vi "ESC controller ramped.vi"(1 "Don't Wait":bool, 2 "Error In":errorcluster, 3 "Output %":sgl min=0 max=100) -> (0 "Error out":errorcluster)   [LabVIEW 2021]
uses:
  Anemometry/Anemometry Sub Vis/Gen Trav/Multi_Run_Status.ctl
  Anemometry/Anemometry Sub Vis/Globals/Meas_global.vi
panel:
  out "Current":dbl
  out "Dem Steps":dbl[](array[numeric])
  in  "Step Size %":dbl=3.0
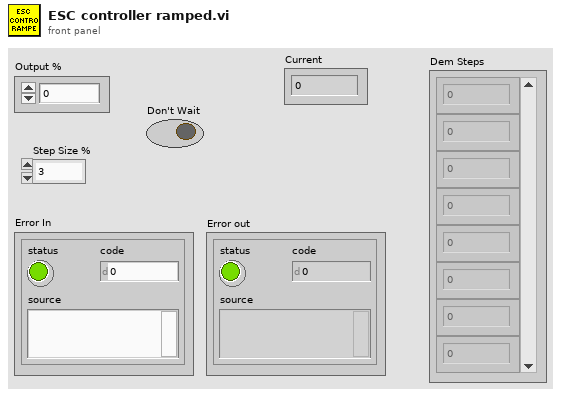
[diagram p1: front panel]
types:
  T1 = typedef "Multi_Run_Status.ctl" = enum16{"Continue", "Continue with Error", "Jump to Next Point", "Jump to Next Row", "Jump To Fall Back", "Terminate Run"}
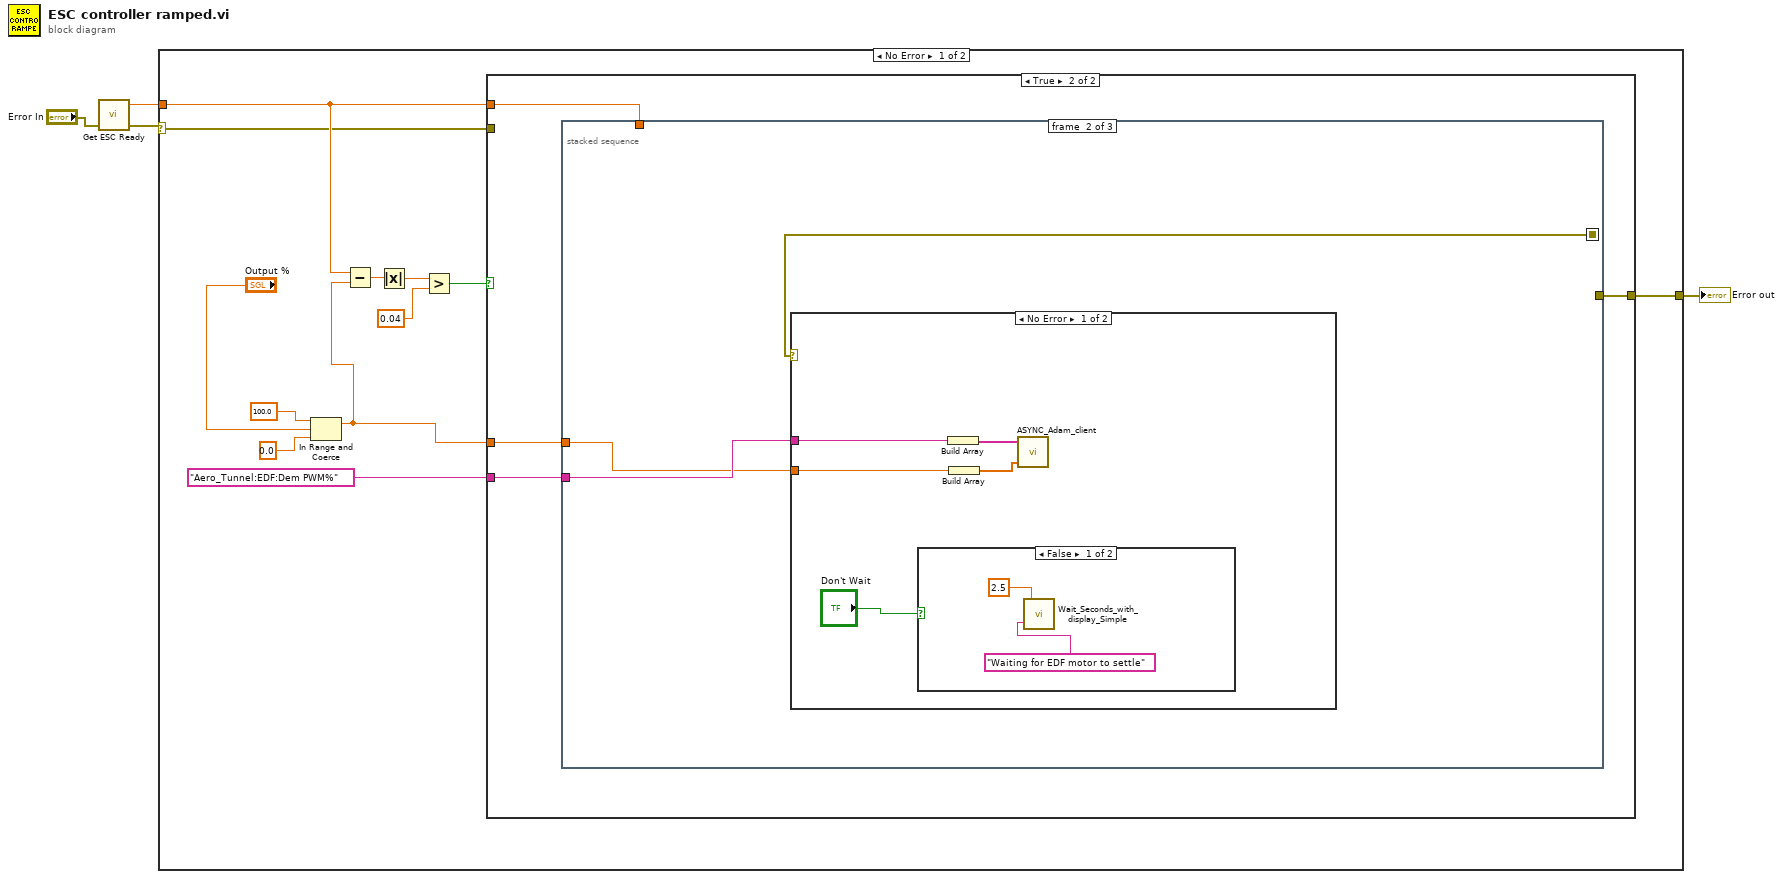
[diagram p0: block diagram]
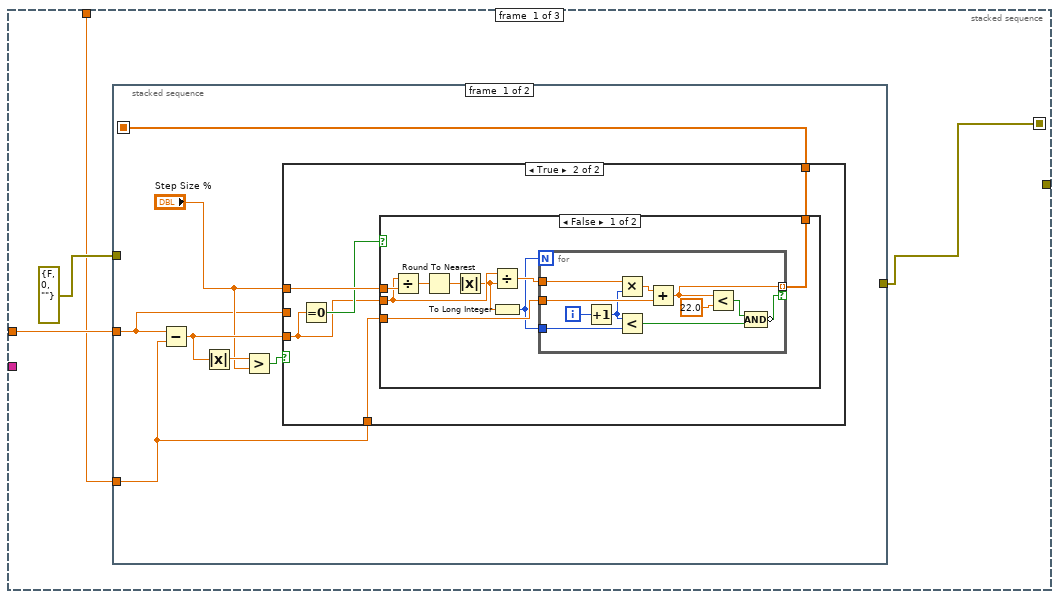
[diagram p3: hidden frame]
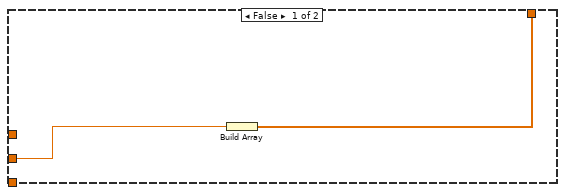
[diagram p4: hidden frame]
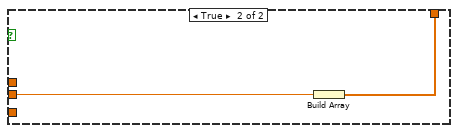
[diagram p5: hidden frame]
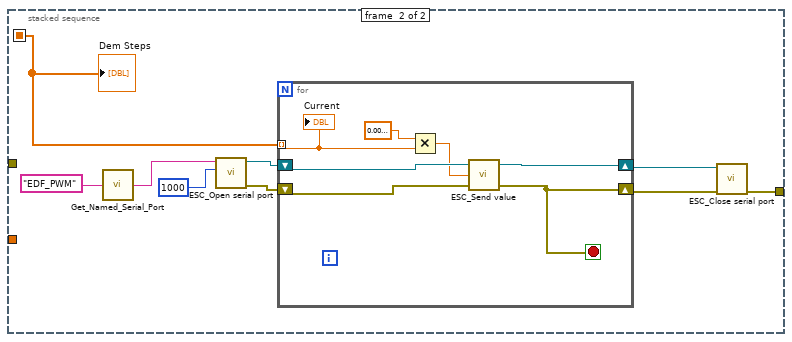
[diagram p6: hidden frame]
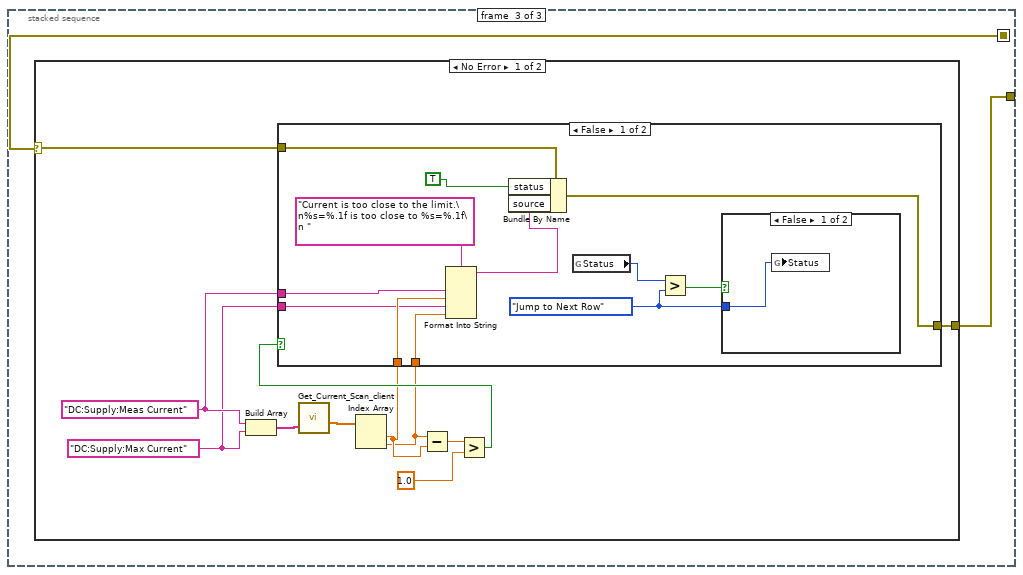
[diagram p9: hidden frame]
diagram:
  n1 = call "Get ESC Ready.vi"("Error in"="Error In") -> ("Error out"=w2:errorcluster, "Current PWM%"=w1:dbl)  [unwired: 3 in]
  n2 = case shown="No Error" w2 {
    selector: w2 -> [w5 w116]
    tunnel: [w15 w116] -> w4
    tunnel: w1 -> [w11 _]
    frame No Error {
      n3 = In Range and Coerce(upper limit=sgl 100.0, x="Output %", lower limit=sgl 0.0) -> (coerced(x)=w10:sgl)  [unwired: 1 out]
      n4 = Subtract(x=w11, y=w10) -> (x-y=w9:dbl)
      n5 = Absolute Value(x=w9) -> (abs(x)=w8:dbl)
      n6 = Greater?(x=w8, y=0.04) -> (0:w6:bool)
      n7 = case shown="True" w6 {
        tunnel: "Aero_Tunnel:EDF:Dem PWM%" -> [_ w21]
        tunnel: [w17 w20] -> w15
        tunnel: w11 -> [_ w19]
        tunnel: w10 -> [_ w18]
        tunnel: w5 -> [w17 _]
        frame False {
        }
        frame True {
          n8 = stacked-sequence {
            seq-local: [w25 _ _] -> [_ w80 w89]
            tunnel: w21 -> [_ w79 _]
            tunnel: w18 -> [w23 w78 _]
            tunnel: [_ _ w88] -> w20
            tunnel: w19 -> [w22 _ _]
            frame #0 {
              n9 = stacked-sequence {
                seq-local: [w31 _] -> [_ w62]
                tunnel: [_ w68] -> w25
                tunnel: errorcluster {"status"=FALSE, "code"=0, "source"=""} ("Error out") -> [_ _]
                tunnel: w22 -> [w32 _]
                tunnel: w23 -> [w26 _]
                frame #0 {
                  n10 = Subtract(x=w26, y=w32) -> (x-y=w30:dbl)
                  n11 = Absolute Value(x=w30) -> (abs(x)=w28:dbl)
                  n12 = Greater?(x=w28, y="Step Size %") -> (0:w29:bool)
                  n13 = case shown="True" w29 {
                    tunnel: "Step Size %" -> [_ w39]
                    tunnel: w32 -> [_ w37]
                    tunnel: [w33 w36] -> w31
                    tunnel: w30 -> [_ w35]
                    tunnel: w26 -> [w34 _]
                    frame False {
                      n14 = Build Array(w34) -> (w33:sgl[])
                    }
                    frame True {
                      n15 = Equal To 0?(x=w35) -> (x = 0?=w38:bool)
                      n16 = case shown="False" w38 {
                        tunnel: w39 -> [w48 _]
                        tunnel: w37 -> [w45 _]
                        tunnel: [w43 w60] -> w36
                        tunnel: w35 -> [w42 w61]
                        frame False {
                          n17 = Divide(x=w42, y=w48) -> (x/y=w47:dbl)
                          n18 = Round To Nearest(number=w47) -> (nearest integer value=w46:dbl)
                          n19 = Absolute Value(x=w46) -> (abs(x)=w41:dbl)
                          n20 = Divide(x=w42, y=w41) -> (x/y=w44:dbl)
                          n21 = To Long Integer(number=w41) -> (32bit integer=w40:i32)
                          n22 = for {
                            N: w40 -> [_]
                            tunnel: w45 -> [w59]
                            tunnel: w44 -> [w57]
                            tunnel: [w55] -> w43 mode=indexing if=w49
                            tunnel: w40 -> [w52]
                            i -> [w58]
                            n23 = Increment(x=w58) -> (x+1=w53:i32)
                            n24 = Multiply(x=w57, y=w53) -> (x*y=w56:dbl)
                            n25 = Less?(x=w53, y=w52) -> (x < y?=w50:bool)
                            n26 = Add(x=w56, y=w59) -> (x+y=w55:dbl)
                            n27 = Less?(x=w55, y=22.0) -> (x < y?=w51:bool)
                            n28 = Compound Arithmetic op=AND(w51, w50) -> (invert w49:bool)
                          }
                        }
                        frame True {
                          n29 = Build Array(w61) -> (w60:dbl[])
                        }
                      }
                    }
                  }
                }
                frame #1 {
                  n30 = call "Get_Named_Serial_Port.vi"("Serial Port Alias"="EDF_PWM") -> ("Serial Port Name"=w70:string)
                  n31 = call "ESC_Open serial port.vi"("timeout (ms)"=u32 1000, "VISA resource name"=w70) -> ("Error out"=w66:errorcluster, "VISA resource name out"=w65:refnum<visa-resource-name>)  [unwired: 8 in]
                  n32 = for {
                    shift-right: [w71] -> w64
                    shift-left: w66 -> [w77]
                    shift-right: [w73] -> w63
                    shift-left: w65 -> [w76]
                    tunnel: w62 -> [w72] mode=indexing
                    stop <- w71 stop-if-true
                    n33 = Multiply(x=sgl 0.01, y=w72) -> (x*y=w75:dbl)
                    n34 = call "ESC_Send value.vi"("Error In"=w77, "Output (0...1)"=w75, "Port"=w76) -> ("Error Out"=w71:errorcluster, "Port out"=w73:refnum<visa-resource-name>)  [unwired: 1 out]
                    "Current" <- w72
                  }
                  n35 = call "ESC_Close serial port.vi"("Error in"=w64, "VISA resource name"=w63) -> ("Error out"=w68:errorcluster)  [unwired: 9 in]
                  "Dem Steps" <- w62
                }
              }
            }
            frame #1 {
              n36 = case shown="No Error" w80 {
                tunnel: w79 -> [w83 _]
                tunnel: w78 -> [w82 _]
                frame No Error {
                  n37 = case shown="False" "Don't Wait" {
                    frame False {
                      n38 = call "Wait_Seconds_with_display_Simple.vi"("Message"="Waiting for EDF motor to settle", "Seconds to wait"=2.5) -> ()  [unwired: 1 in, 1 out]
                    }
                    frame True {
                    }
                  }
                  n39 = Build Array(w83) -> (w85:string[])
                  n40 = Build Array(w82) -> (w84:sgl[])
                  n41 = call "ASYNC_Adam_client.vi"("Values"=w84, "Channel Names"=w85) -> ()  [unwired: 1 in, 2 out]
                }
                frame Error {
                }
              }
            }
            frame #2 {
              n42 = case shown="No Error" w89 {
                selector: w89 -> [w94 w115]
                tunnel: [w95 w115] -> w88
                frame No Error {
                  w91 = "DC:Supply:Max Current" ("string")
                  w93 = "DC:Supply:Meas Current"
                  n43 = Build Array(w93, w91) -> (w100:string[])
                  n44 = call "Get_Current_Scan_client.vi"("multipleChannels"=w100) -> ("Numerical Values"=w99:dbl[])  [unwired: 1 in, 3 out]
                  n45 = Index Array(array=w99) -> (element #1=w92:dbl, element #2=w90:dbl)  [unwired: 2 in]
                  n46 = Subtract(x=w90, y=w92) -> (x-y=w98:dbl)
                  n47 = Greater?(x=w98, y=1.0) -> (0:w96:bool)
                  n48 = case shown="False" w96 {
                    tunnel: [w104 w114] -> w95
                    tunnel: w94 -> [w112 w114]
                    tunnel: w93 -> [w109 _]
                    tunnel: w92 -> [w110 _]
                    tunnel: w91 -> [w108 _]
                    tunnel: w90 -> [w107 _]
                    frame False {
                      w101 = Multi_Run_Status."Jump to Next Row" ("Status")
                      n49 = Format Into String(format string="Current is too close to the limit.\n%s=%.1f is too close to %s=%.1f\n ", w109, w110, w108, w107) -> (resulting string=w105:string)  [unwired: 2 in, 1 out]
                      n50 = Bundle By Name(cluster=w112, "status"=TRUE, "source"=w105) -> (w104:errorcluster)
                      n51 = global read "Meas_global.vi" "Status"() -> (w103:T1)
                      n52 = Greater?(x=w103, y=w101) -> (0:w102:bool)
                      n53 = case shown="False" w102 {
                        tunnel: w101 -> [w113 _]
                        frame False {
                          n54 = global write "Meas_global.vi" "Status"(w113) -> ()
                        }
                        frame True {
                        }
                      }
                    }
                    frame True {
                    }
                  }
                }
                frame Error {
                }
              }
            }
          }
        }
      }
    }
    frame Error {
    }
  }
  "Error out" <- w4
